vi "test placeholder.vi"() -> ()   [LabVIEW 2013]
panel:
  out "pass?":bool
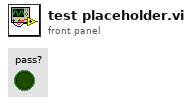
[diagram p1: front panel]
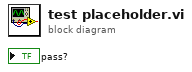
[diagram p0: block diagram]
diagram:
